vi "Write Dict.vi"(8 "error in (no error)":errorcluster, 10 "Dict":variant, 11 "Dictionary in":refnum<class "Dictionary.lvclass">) -> (0 "error out":errorcluster, 3 "Dictionary out":refnum<class "Dictionary.lvclass">)   [LabVIEW 2014, in "bmlv.lvlib" / "Dictionary.lvclass"]
uses:
  Dictionary.lvclass
  Dictionary.lvclass/Dictionary.ctl
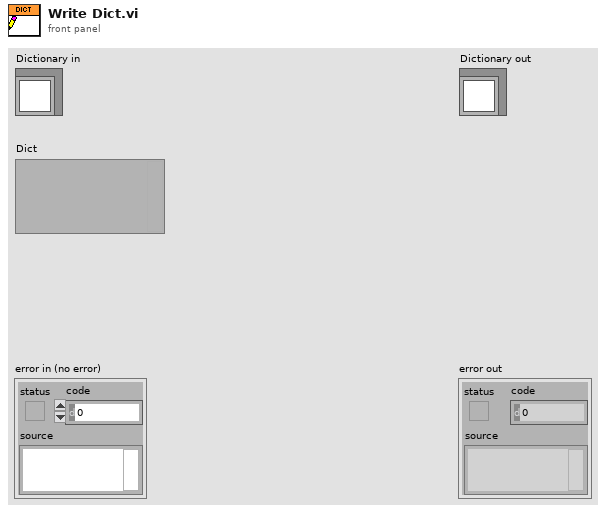
[diagram p1: front panel]
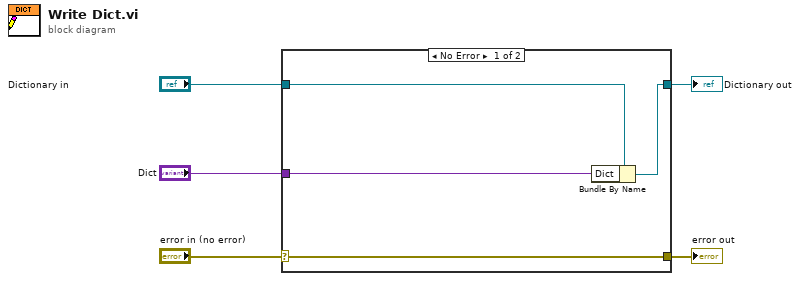
[diagram p0: block diagram]
diagram:
  n1 = case shown="No Error" "error in (no error)" {
    selector: "error in (no error)" -> [w9 w10]
    tunnel: [w9 w10] -> w4
    tunnel: [w7 w11] -> w2
    tunnel: "Dictionary in" -> [w8 w11]
    tunnel: "Dict" -> [w6 _]
    frame No Error {
      n2 = Bundle By Name(cluster=w8, "Dict"=w6) -> (w7:refnum<class "Dictionary.lvclass">)
    }
    frame Error {
    }
  }
  "error out" <- w4
  "Dictionary out" <- w2
